vi "U8ToU32.vi"(4 "Index":u32, 7 "Input U8 Array":u8[](array[numeric])) -> (0 "Index+4":u32, 1 "Output U32":u32, 3 "Output U8 Array":u8[](array[numeric]))   [LabVIEW 2017]
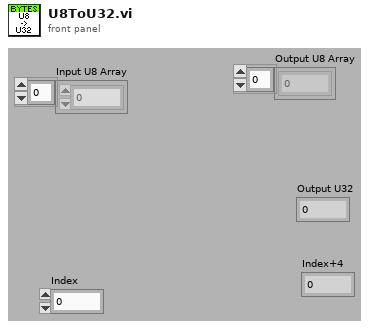
[diagram p1: front panel]
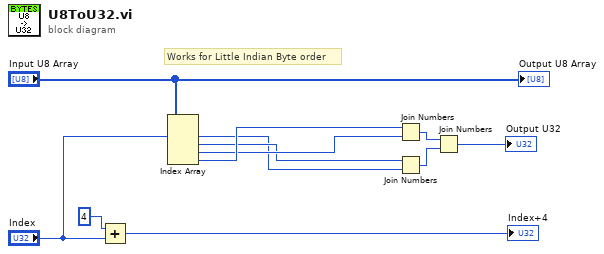
[diagram p0: block diagram]
diagram:
  # "Works for Little Indian Byte order"
  n1 = Add(x=4 ("count (1)"), y="Index") -> (x+y=→"Index+4":u32)
  n2 = Index Array(array="Input U8 Array", index #1="Index") -> (element #1=w4:u8, element #2=w5:u8, element #3=w6:u8, element #4=w7:u8)  [unwired: 3 in]
  n3 = Join Numbers(hi=w7, lo=w6) -> ((hi.lo)=w9:u16)
  n4 = Join Numbers(hi=w5, lo=w4) -> ((hi.lo)=w8:u16)
  n5 = Join Numbers(hi=w9, lo=w8) -> ((hi.lo)=→"Output U32":u32)
  "Output U8 Array" <- "Input U8 Array"
